vi "Load Configuration.vi"(8 "error in":errorcluster, 11 "Configuration File":path) -> (0 "error out":errorcluster, 1 "Data Directory":path, 2 "Microphone Locations":cluster{"r":dbl, "theta":dbl, "z":dbl}[](array[cluster]), 3 "DAQ Channels":string)   [LabVIEW 2013, in "Breakdown Acoustics Controls.lvlib"]
uses:
  <vilib>/xml/Load XML File.vi
  <vilib>/xml/Close Reference(Node).vi
  Breakdown Acoustics Controls.lvlib
  <vilib>/xml/NI_XML.lvlib
  <resource>/objmgr/DOMUserDefRef.rc
panel:
  out "parse errors":string
  in  "Transducer Coordinates (cm, rad)":cluster{"r":dbl, "theta":dbl}[](array[cluster])
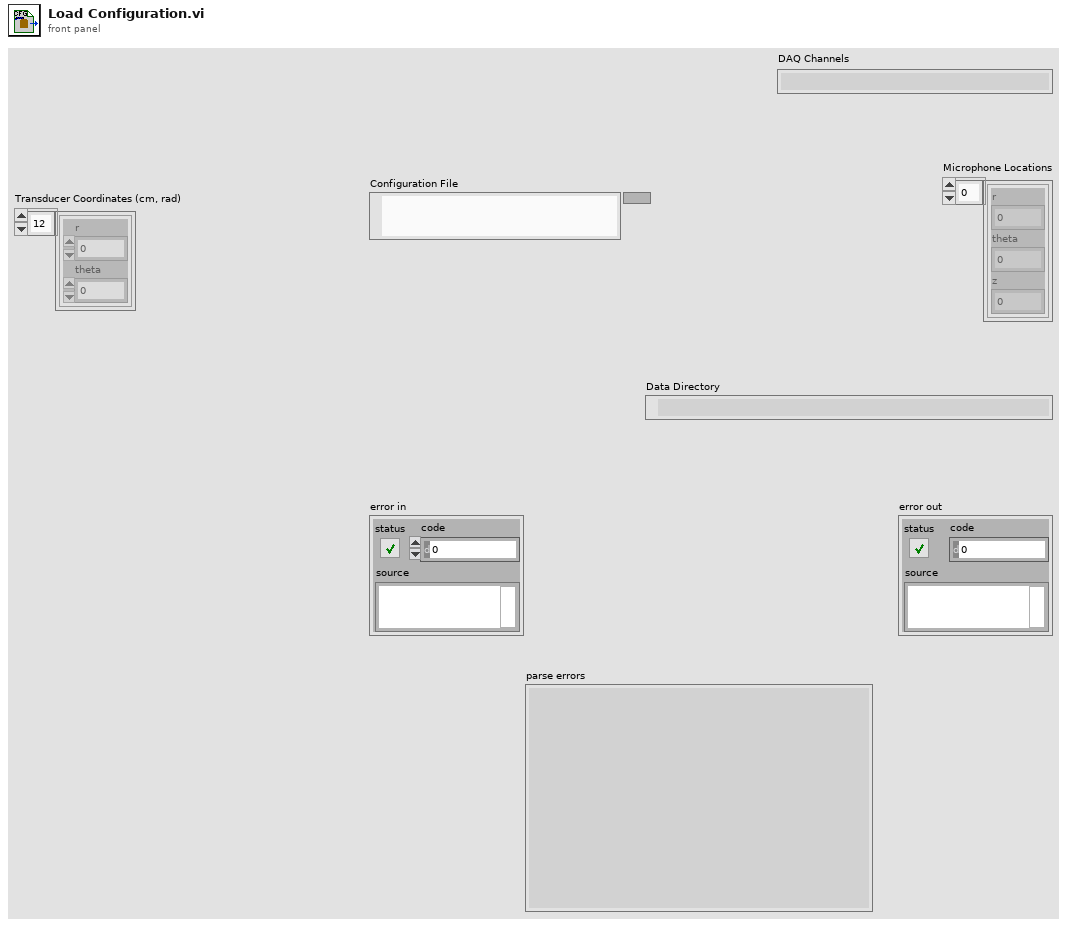
[diagram p1: front panel]
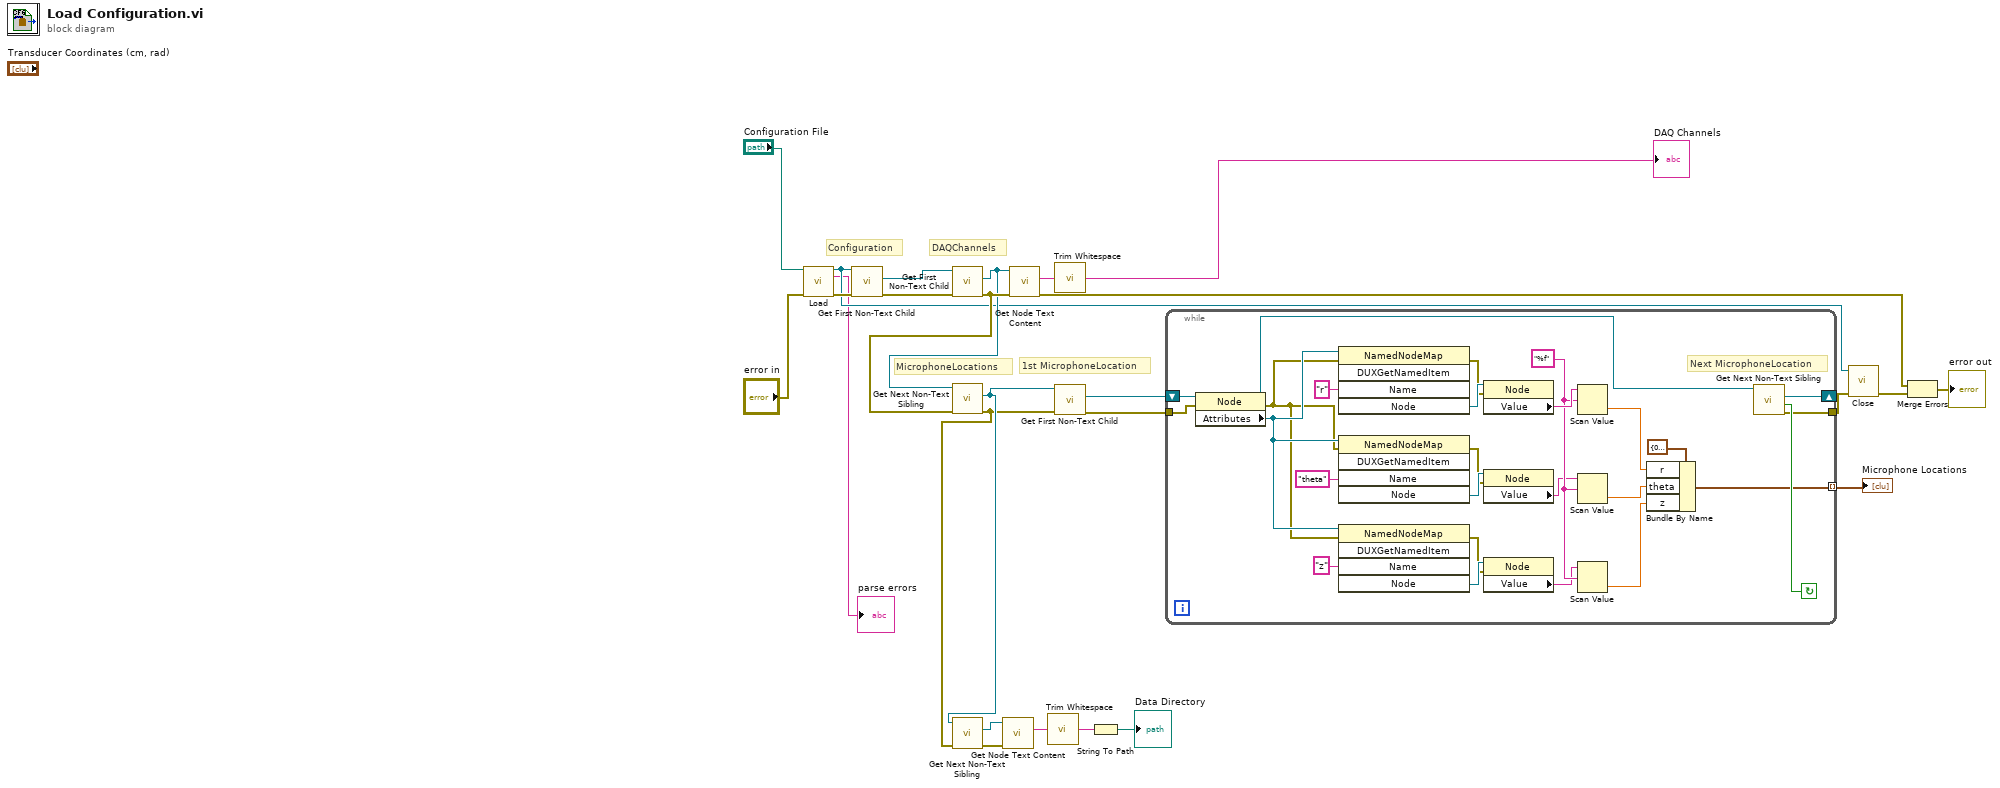
[diagram p0: block diagram]
diagram:
  # "1st MicrophoneLocation"
  # "MicrophoneLocations"
  # "DAQChannels"
  # "Configuration"
  n1 = call-poly <vilib>:"Load.vi"("path to XML document"="Configuration File", "error in (no error)"="error in") -> ("DOM document out"=w13:refnum<k20>, "parse errors"=→"parse errors":string, "error out"=w23:errorcluster)  [unwired: 11 in]
  n2 = call <vilib>:"Get First Non-Text Child.vi"("error in (no error)"=w23, "node in"=w13) -> ("error out"=w22:errorcluster, "child node"=w11:refnum<k20>)  [unwired: 6 in, 2 out]
  n3 = call <vilib>:"Get First Non-Text Child.vi"("error in (no error)"=w22, "node in"=w11) -> ("error out"=w19:errorcluster, "child node"=w14:refnum<k20>)  [unwired: 6 in, 2 out]
  n4 = call <vilib>:"Get Next Non-Text Sibling.vi"("error in (no error)"=w19, "node in"=w14) -> ("error out"=w6:errorcluster, "sibling node"=w7:refnum<k20>)  [unwired: 6 in, 2 out]
  n5 = call <vilib>:"Get Next Non-Text Sibling.vi"("error in (no error)"=w6, "node in"=w7) -> ("error out"=w3:errorcluster, "sibling node"=w4:refnum<k20>)  [unwired: 6 in, 2 out]
  n6 = call <vilib>:"Get Node Text Content.vi"("error in (no error)"=w3, "node in"=w4) -> ("node text"=w5:string)  [unwired: 7 in, 2 out]
  n7 = call <vilib>:"Get Node Text Content.vi"("error in (no error)"=w19, "node in"=w14) -> ("error out"=w17:errorcluster, "node text"=w10:string)  [unwired: 7 in, 1 out]
  n8 = call <vilib>:"Trim Whitespace.vi"("string"=w5) -> ("trimmed string"=w2:string)  [unwired: 1 in]
  n9 = call <vilib>:"Trim Whitespace.vi"("string"=w10) -> ("trimmed string"=→"DAQ Channels":string)  [unwired: 1 in]
  n10 = call <vilib>:"Get First Non-Text Child.vi"("error in (no error)"=w6, "node in"=w7) -> ("error out"=w21:errorcluster, "child node"=w20:refnum<k20>)  [unwired: 6 in, 2 out]
  n11 = String To Path(string=w2) -> (path=→"Data Directory":path)
  n12 = while {
    tunnel: w21 -> [w47]
    shift-right: [w50] -> _
    shift-left: w20 -> [w48]
    tunnel: [w49] -> w16
    tunnel: [w27] -> w8 mode=indexing
    stop <- w51 continue-if-true
    w34 = "%f" ("format string")
    # "Next MicrophoneLocation"
    n13 = property class="Node"(reference=w48, error in=w47) -> (reference out=w26:refnum<k20>, error out=w42:errorcluster, "Attributes"=w43:refnum<k20>)
    n14 = invoke class="NamedNodeMap" method="DUXGetNamedItem"(reference=w43, error in=w42, "Name"="r") -> (error out=w36:errorcluster, "Node"=w41:refnum<k20>)  [unwired: 2 in, 3 out]
    n15 = invoke class="NamedNodeMap" method="DUXGetNamedItem"(reference=w43, error in=w42, "Name"="theta") -> (error out=w37:errorcluster, "Node"=w40:refnum<k20>)  [unwired: 2 in, 3 out]
    n16 = invoke class="NamedNodeMap" method="DUXGetNamedItem"(reference=w43, error in=w42, "Name"="z") -> (error out=w38:errorcluster, "Node"=w39:refnum<k20>)  [unwired: 2 in, 3 out]
    n17 = property class="Node"(reference=w41, error in=w36) -> ("Value"=w35:string)  [unwired: 2 out]
    n18 = property class="Node"(reference=w40, error in=w37) -> ("Value"=w33:string)  [unwired: 2 out]
    n19 = property class="Node"(reference=w39, error in=w38) -> ("Value"=w32:string)  [unwired: 2 out]
    n20 = Scan Value(string=w35, format string=w34) -> (value=w30:dbl)  [unwired: 1 in, 1 out]
    n21 = Scan Value(string=w33, format string=w34) -> (value=w29:dbl)  [unwired: 1 in, 1 out]
    n22 = Scan Value(string=w32, format string=w34) -> (value=w28:dbl)  [unwired: 1 in, 1 out]
    n23 = Bundle By Name(cluster=cluster{"r":dbl, "theta":dbl, "z":dbl} {"r"=0.0, "theta"=0.0, "z"=0.0} ("Polar\nCoordinates"), "r"=w30, "theta"=w29, "z"=w28) -> (w27:cluster{"r":dbl, "theta":dbl, "z":dbl})
    n24 = call <vilib>:"Get Next Non-Text Sibling.vi"("node in"=w26) -> ("error out"=w49:errorcluster, "found sibling node?"=w51:bool, "sibling node"=w50:refnum<k20>)  [unwired: 7 in, 1 out]
  }
  "Microphone Locations" <- w8
  n25 = call-poly <vilib>:"Close.vi"("error in (no error)"=w16, "node"=w13) -> ("error out"=w15:errorcluster)  [unwired: 7 in]
  n26 = Merge Errors(w17, w15) -> (→"error out":errorcluster)
